vi "TestLEDS.vi"(9 "Time(ms)":u32, 10 "枚举":T1(ring), 11 "TestIndex":i32) -> (1 "FLASH DATA":i32[](array[numeric]), 2 "数值":i32)   [LabVIEW 2015]
uses:
  Global variable.vi
panel:
  out "数组 4":i32[][](array[numeric])
  out "数组 3":i32[](array[numeric])
  out "数组 2":bool[][](array[boolean])
  out "字符串":string
  out "数组":i32[](array[numeric])
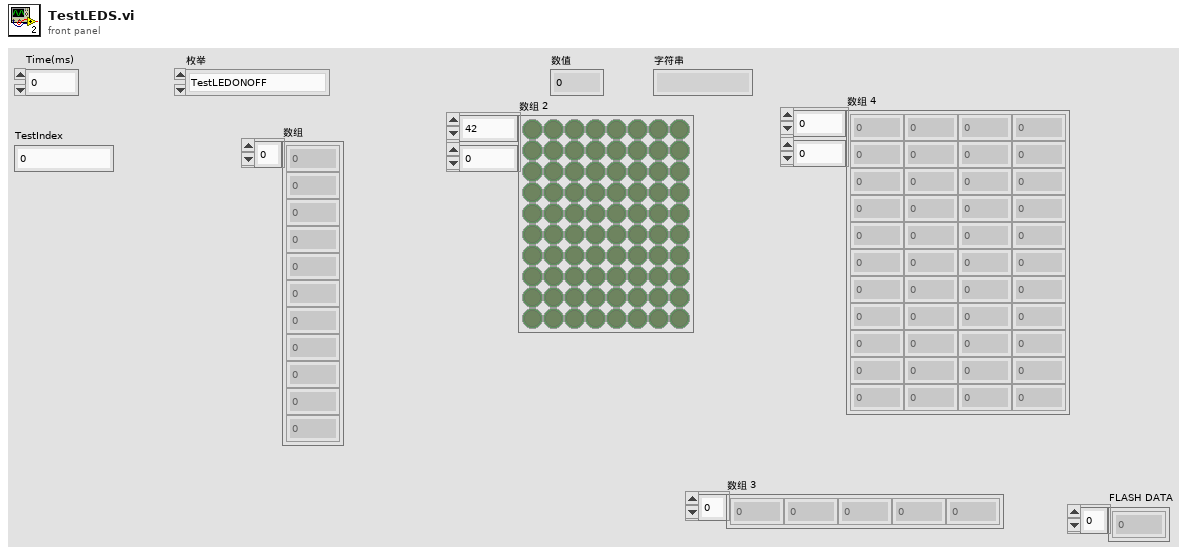
[diagram p1: front panel]
types:
  T1 = enum16{"TestLEDONOFF", "TestLEDFlash", "TestVersion"}
  T2 = cluster{"CH1603":refnum<visa-resource-name>, "VSMD124_025T":refnum<visa-resource-name>, "RPM表":refnum<visa-resource-name>, "ACSource安姆泰克":refnum<visa-resource-name>, "VICTOR8246":refnum<visa-resource-name>, "MSP-Gang":refnum<visa-resource-name>, "6724Power":refnum<visa-resource-name>, "electric load":refnum<visa-resource-name>, "Arduino":refnum<visa-resource-name>}
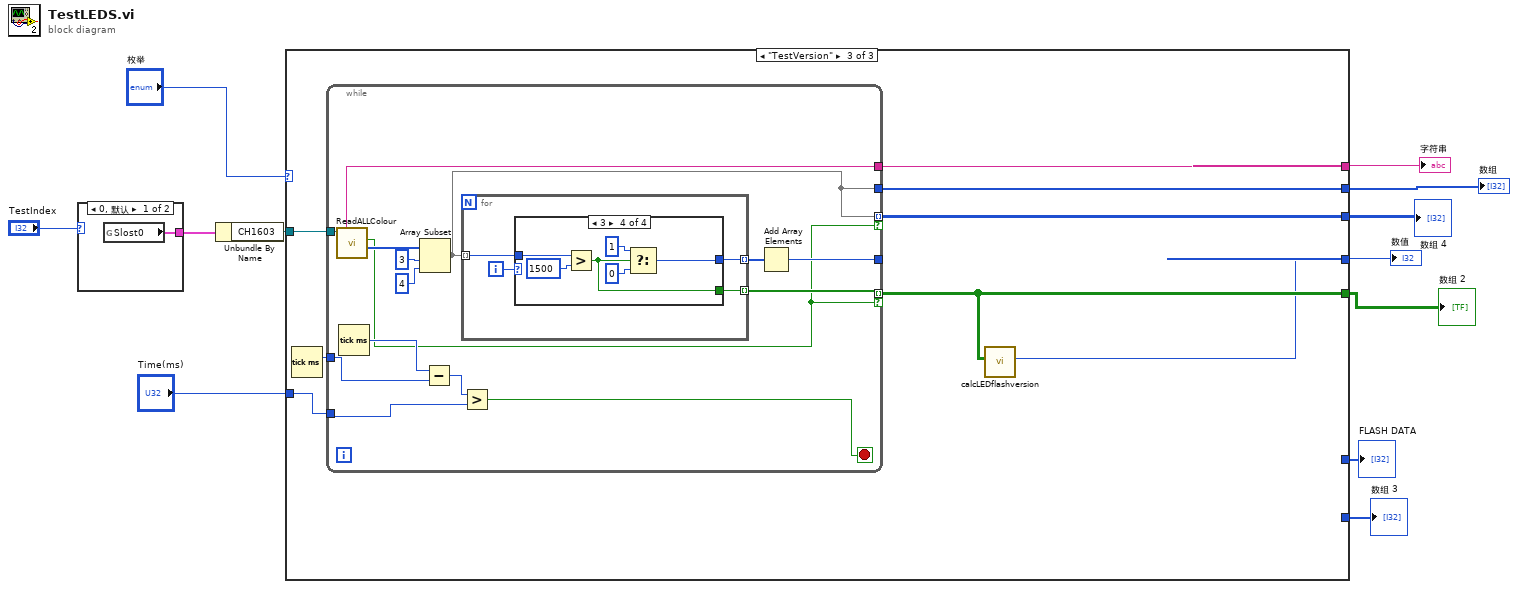
[diagram p0: block diagram]
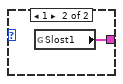
[diagram p2: hidden frame]
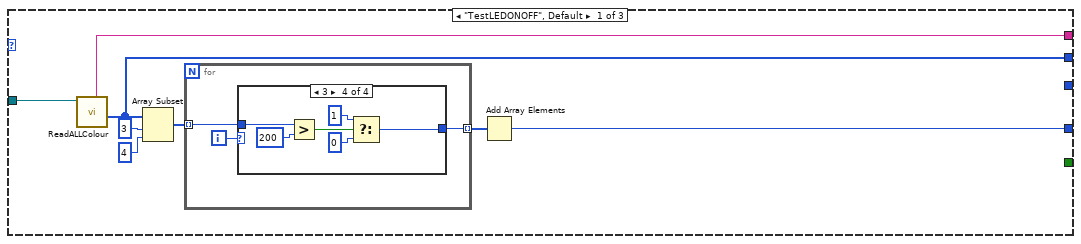
[diagram p3: hidden frame]
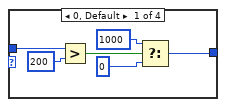
[diagram p4: hidden frame]
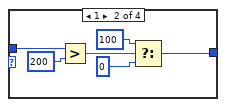
[diagram p5: hidden frame]
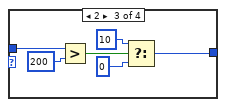
[diagram p6: hidden frame]
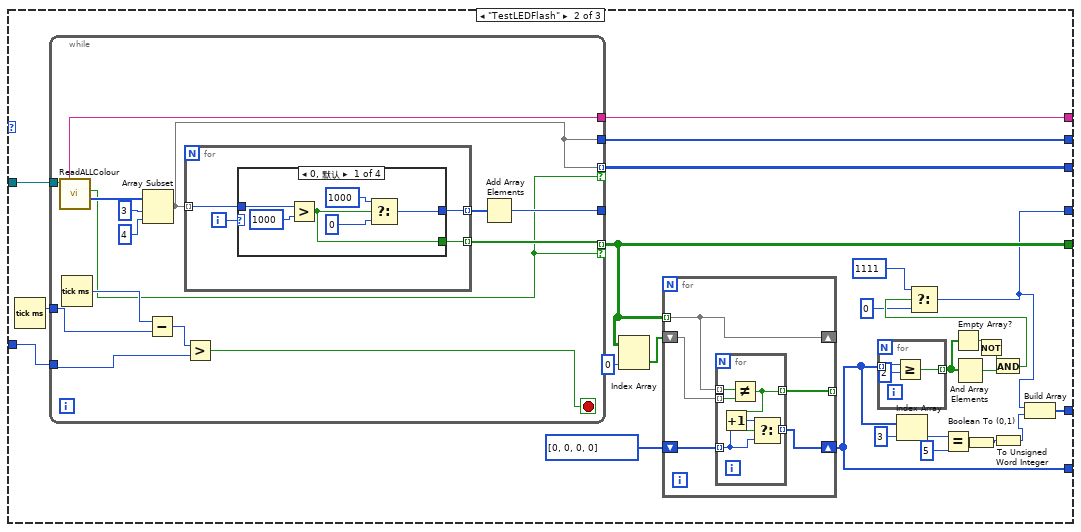
[diagram p7: hidden frame]
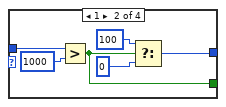
[diagram p8: hidden frame]
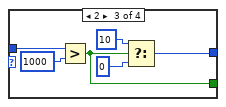
[diagram p9: hidden frame]
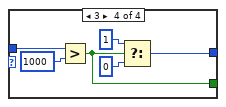
[diagram p10: hidden frame]
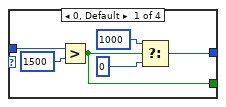
[diagram p11: hidden frame]
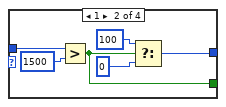
[diagram p12: hidden frame]
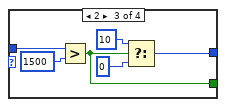
[diagram p13: hidden frame]
diagram:
  n1 = case shown="0, 默认" "TestIndex" {
    tunnel: [w13 w14] -> w11
    frame 0, Default {
      n2 = global read "Global variable.vi" "Slost0"() -> (w13:T2)
    }
    frame 1 {
      n3 = global read "Global variable.vi" "Slost1"() -> (w14:T2)
    }
  }
  n4 = Unbundle By Name(w11) -> ("CH1603"=w10:refnum<visa-resource-name>)
  n5 = case shown="\"TestVersion\"" "枚举" {
    tunnel: w10 -> [w22 w75 w140]
    tunnel: [w17 w53 w133] -> w8
    tunnel: [w16 w74 w139] -> w7
    tunnel: [w15 w73 w138] -> w6
    tunnel: "Time(ms)" -> [_ w71 w136]
    tunnel: [_ w70 w134] -> w4
    tunnel: [_ w66 w135] -> w3
    tunnel: [_ w58 _] -> w2
    tunnel: [_ w51 _] -> w1
    frame "TestLEDONOFF", Default {
      n6 = call "ReadALLColour.vi"("CH1603"=w22) -> ("数组"=w16:i32[], "字符串"=w15:string)  [unwired: 8 in, 1 out]
      n7 = Array Subset(array=w16, index=3 ("索引"), length=4 ("长度")) -> (w19:i32[])
      n8 = for {
        tunnel: w19 -> [w24] mode=indexing
        tunnel: [w23] -> w18 mode=indexing
        i -> [w25]
        n9 = case shown="3" w25 {
          tunnel: w24 -> [w31 w37 w43 w49]
          tunnel: [w26 w32 w38 w44] -> w23
          frame 0, Default {
            n10 = Greater?(x=w31, y=200) -> (0:w29:bool)
            n11 = Select(t=1000, s=w29, f=0) -> (s? t:f=w26:i32)
          }
          frame 1 {
            n12 = Greater?(x=w37, y=200) -> (0:w35:bool)
            n13 = Select(t=100, s=w35, f=0) -> (s? t:f=w32:i32)
          }
          frame 2 {
            n14 = Greater?(x=w43, y=200) -> (0:w41:bool)
            n15 = Select(t=10, s=w41, f=0) -> (s? t:f=w38:i32)
          }
          frame 3 {
            n16 = Greater?(x=w49, y=200) -> (0:w47:bool)
            n17 = Select(t=1, s=w47, f=0) -> (s? t:f=w44:i32)
          }
        }
      }
      n18 = Add Array Elements(numeric array=w18) -> (sum=w17:i32)
    }
    frame "TestLEDFlash" {
      n19 = Tick Count (ms)() -> (millisecond timer value=w72:u32)
      n20 = while {
        tunnel: w75 -> [w104]
        tunnel: [w103] -> _
        tunnel: [w91] -> w74
        tunnel: [w102] -> w73
        tunnel: w72 -> [w94]
        tunnel: w71 -> [w100]
        tunnel: [w96] -> w70 mode=indexing if=w90
        tunnel: [w91] -> w66 mode=indexing if=w90
        stop <- w95 stop-if-true
        n21 = call "ReadALLColour.vi"("CH1603"=w104) -> ("数组"=w92:i32[], "布尔"=w90:bool, "字符串"=w102:string)  [unwired: 8 in]
        n22 = Tick Count (ms)() -> (millisecond timer value=w93:u32)
        n23 = Array Subset(array=w92, index=3 ("索引"), length=4 ("长度")) -> (w91:i32[])
        n24 = Subtract(x=w93, y=w94) -> (x-y=w101:u32)
        n25 = for {
          tunnel: w91 -> [w107] mode=indexing
          tunnel: [w106] -> w97 mode=indexing
          tunnel: [w105] -> w96 mode=indexing
          i -> [w108]
          n26 = case shown="0, 默认" w108 {
            tunnel: w107 -> [w114 w120 w126 w132]
            tunnel: [w110 w116 w122 w128] -> w106
            tunnel: [w109 w115 w121 w127] -> w105
            frame 0, Default {
              n27 = Greater?(x=w114, y=1000) -> (0:w109:bool)
              n28 = Select(t=1000, s=w109, f=0) -> (s? t:f=w110:i32)
            }
            frame 1 {
              n29 = Greater?(x=w120, y=1000) -> (0:w115:bool)
              n30 = Select(t=100, s=w115, f=0) -> (s? t:f=w116:i32)
            }
            frame 2 {
              n31 = Greater?(x=w126, y=1000) -> (0:w121:bool)
              n32 = Select(t=10, s=w121, f=0) -> (s? t:f=w122:i32)
            }
            frame 3 {
              n33 = Greater?(x=w132, y=1000) -> (0:w127:bool)
              n34 = Select(t=1, s=w127, f=0) -> (s? t:f=w128:i32)
            }
          }
        }
        n35 = Greater?(x=w101, y=w100) -> (0:w95:bool)
        n36 = Add Array Elements(numeric array=w97) -> (sum=w103:i32)
      }
      n37 = Index Array(array=w70, index (row)=0 ("索引 (行)")) -> (element=w68:bool[])  [unwired: 1 in]
      n38 = for {
        tunnel: w70 -> [w83] mode=indexing
        shift-right: [w83] -> _
        shift-left: w68 -> [w82]
        tunnel: [w81] -> _ mode=indexing
        shift-right: [w79] -> w58
        shift-left: i32[] [0, 0, 0, 0] -> [w80]
        n39 = for {
          tunnel: w83 -> [w88] mode=indexing
          tunnel: w82 -> [w89] mode=indexing
          tunnel: [w87] -> w81 mode=indexing
          tunnel: w80 -> [w85] mode=indexing
          tunnel: [w84] -> w79 mode=indexing
          n40 = Increment(x=w85) -> (x+1=w86:i32)
          n41 = Not Equal?(x=w88, y=w89) -> (x != y?=w87:bool)
          n42 = Select(t=w86, s=w87, f=w85) -> (s? t:f=w84:i32)
        }
      }
      n43 = for {
        tunnel: w58 -> [w78] mode=indexing
        tunnel: [w76] -> w64 mode=indexing
        n44 = Greater Or Equal?(x=w78, y=2) -> (x >= y?=w76:bool)
      }
      n45 = Index Array(array=w58, index=3 ("索引")) -> (element=w56:i32)
      n46 = Equal?(x=w56, y=5) -> (x = y?=w54:bool)
      n47 = Empty Array?(array=w64) -> (empty?=w63:bool)
      n48 = And Array Elements(Boolean array=w64) -> (logical AND=w65:bool)
      n49 = Boolean To (0,1)(Boolean=w54) -> (0, 1=w52:i16)
      n50 = Not(x=w63) -> (.not. x?=w62:bool)
      n51 = And(x=w62, y=w65) -> (x .and. y?=w61:bool)
      n52 = Select(t=u16 1111, s=w61, f=0) -> (s? t:f=w53:i32)
      n53 = To Unsigned Word Integer(number=w52) -> (unsigned 16bit integer=w50:u16)
      n54 = Build Array(w53, w50) -> (w51:i32[])
    }
    frame "TestVersion" {
      n55 = Tick Count (ms)() -> (millisecond timer value=w137:u32)
      n56 = while {
        tunnel: w140 -> [w155]
        tunnel: [w154] -> _
        tunnel: [w142] -> w139
        tunnel: [w153] -> w138
        tunnel: w137 -> [w145]
        tunnel: w136 -> [w151]
        tunnel: [w147] -> w134 mode=indexing if=w141
        tunnel: [w142] -> w135 mode=indexing if=w141
        stop <- w146 stop-if-true
        n57 = call "ReadALLColour.vi"("CH1603"=w155) -> ("数组"=w143:i32[], "布尔"=w141:bool, "字符串"=w153:string)  [unwired: 8 in]
        n58 = Tick Count (ms)() -> (millisecond timer value=w144:u32)
        n59 = Array Subset(array=w143, index=3 ("索引"), length=4 ("长度")) -> (w142:i32[])
        n60 = Subtract(x=w144, y=w145) -> (x-y=w152:u32)
        n61 = for {
          tunnel: w142 -> [w158] mode=indexing
          tunnel: [w157] -> w148 mode=indexing
          tunnel: [w156] -> w147 mode=indexing
          i -> [w159]
          n62 = case shown="3" w159 {
            tunnel: w158 -> [w165 w171 w177 w183]
            tunnel: [w161 w167 w173 w179] -> w157
            tunnel: [w160 w166 w172 w178] -> w156
            frame 0, Default {
              n63 = Greater?(x=w165, y=1500) -> (0:w160:bool)
              n64 = Select(t=1000, s=w160, f=0) -> (s? t:f=w161:i32)
            }
            frame 1 {
              n65 = Greater?(x=w171, y=1500) -> (0:w166:bool)
              n66 = Select(t=100, s=w166, f=0) -> (s? t:f=w167:i32)
            }
            frame 2 {
              n67 = Greater?(x=w177, y=1500) -> (0:w172:bool)
              n68 = Select(t=10, s=w172, f=0) -> (s? t:f=w173:i32)
            }
            frame 3 {
              n69 = Greater?(x=w183, y=1500) -> (0:w178:bool)
              n70 = Select(t=1, s=w178, f=0) -> (s? t:f=w179:i32)
            }
          }
        }
        n71 = Greater?(x=w152, y=w151) -> (0:w146:bool)
        n72 = Add Array Elements(numeric array=w148) -> (sum=w154:i32)
      }
      n73 = call "calcLEDflashversion.vi"("数组 2"=w134) -> ("数值"=w133:i32)  [unwired: 10 in]
    }
  }
  "数值" <- w8
  "数组" <- w7
  "字符串" <- w6
  "数组 2" <- w4
  "数组 4" <- w3
  "数组 3" <- w2
  "FLASH DATA" <- w1
